vi "Control Shooter.vi"(11 "Avoid Race Condition":bool) -> ()   [LabVIEW 2020]
uses:
  Framework/Robot Global Data.vi
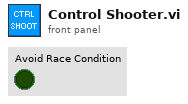
[diagram p1: front panel]
types:
  T1 = typedef "Command Status Info.ctl" = cluster{"Name":string, "Status":T2, "notifier out":T3}
  T2 = typedef "Completion Status.ctl" = enum16{"Successful", "Aborted", "Incomplete"}
  T3 = typedef "Completion Notifier.ctl" = refnum<notifier>
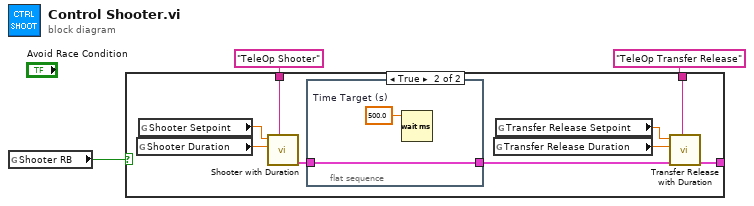
[diagram p0: block diagram]
diagram:
  n1 = global read "Robot Global Data.vi" "Shooter RB"() -> (w1:bool)
  n2 = case shown="True" w1 {
    tunnel: "TeleOp Shooter" ("Description") -> [_ w12]
    tunnel: [_ w9] -> _
    tunnel: "TeleOp Transfer Release" ("Description") -> [_ w8]
    frame False {
    }
    frame True {
      n3 = global read "Robot Global Data.vi" "Shooter Duration"() -> (w10:dbl)
      n4 = global read "Robot Global Data.vi" "Shooter Setpoint"() -> (w11:dbl)
      n5 = call "Shooter with Duration.vi"("Description"=w12, "Duration (s)"=w10, "Setpoint"=w11) -> ("Command Info Out"=w5:T1)  [unwired: 8 in]
      n6 = flat-sequence {
        tunnel: [w13] -> w4
        tunnel: w5 -> [w13]
        frame #0 {
          w14 = 500.0  # Time Target (s)
          n7 = Wait (ms)(milliseconds to wait=w14) -> ()  [unwired: 1 out]
        }
      }
      n8 = global read "Robot Global Data.vi" "Transfer Release Duration"() -> (w7:dbl)
      n9 = global read "Robot Global Data.vi" "Transfer Release Setpoint"() -> (w6:dbl)
      n10 = call "Transfer Release with Duration.vi"("Description"=w8, "Command Info In"=w4, "Duration (s)"=w7, "Setpoint"=w6) -> ("Command Info Out"=w9:T1)  [unwired: 7 in]
    }
  }
